vi "Add block to buffer.vi"(0 "Ring Buffer":T2, 1 "Time Stamp":timestamp, 2 "output type order":T4[](array[typedef]), 5 "data table in":T3, 7 "cache in":T1, 9 "Block size":u16, 11 "error in (no error)":errorcluster, 12 "sample counter in":i32, 13 "Pre-trigger samples?":bool) -> (4 "Ring Buffer out":T2, 6 "data table out":T3, 8 "cache out":T1, 14 "Sample counter out":i32, 15 "error out":errorcluster)   [LabVIEW 2013, in "TDMS datalogger runtime.lvclass"]
uses:
  TDMS datalogger runtime.lvclass
  data cache.ctl
  <vilib>/NI/Tag Bus/table/data table.ctl
  <vilib>/NI/Tag Bus/tag/Data Type.ctl
  Ring Buffer.ctl
  <vilib>/NI/Tag Bus/table/data table.lvlib
  <vilib>/NI/Tag Bus/tag/tag descriptor.lvclass
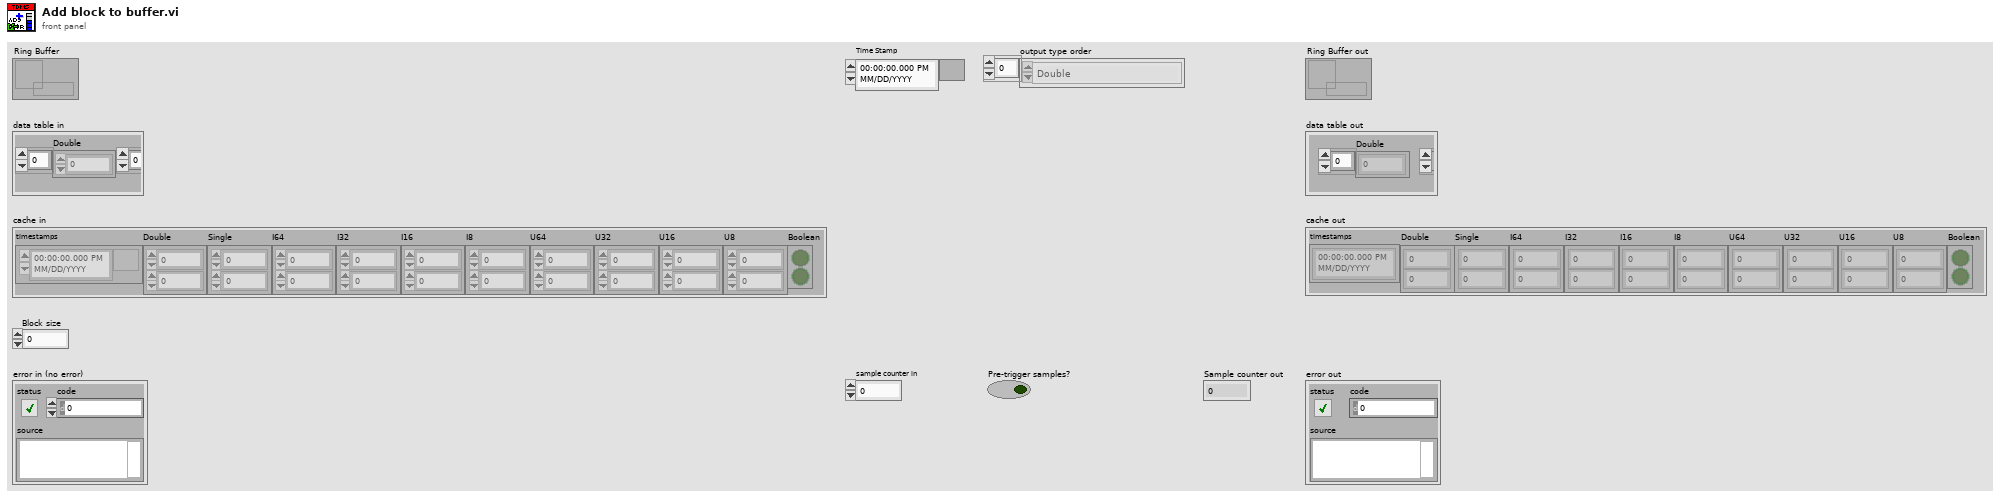
[diagram p1: front panel]
types:
  T1 = typedef "TDMS datalogger runtime.lvclass/data cache.ctl" = cluster{"timestamps":timestamp[], "Double":dbl[][], "Single":sgl[][], "I64":i64[][], "I32":i32[][], "I16":i16[][], "I8":i8[][], "U64":u64[][], "U32":u32[][], "U16":u16[][], "U8":u8[][], "Boolean":bool[][]}
  T2 = typedef "TDMS datalogger runtime.lvclass/Ring Buffer.ctl" = refnum<queue>
  T3 = typedef "tag bus.lvlib/data table.lvlib/data table.ctl" = cluster{"Double":dbl[], "Single":sgl[], "I64":i64[], "I32":i32[], "I16":i16[], "I8":i8[], "U64":u64[], "U32":u32[], "U16":u16[], "U8":u8[], "Boolean":bool[], "String":string[], "Array of Double":cluster{"DBL Array":dbl[]}[], "Array of Single":cluster{"SGL Array":sgl[]}[], "Array of I64":cluster{"I64 Array":i64[]}[], "Array of I32":cluster{"I32 Array":i32[]}[], "Array of I16":cluster{"I16 Array":i16[]}[], "Array of I8":cluster{"I8 Array":i8[]}[], "Array of U64":cluster{"U64 Array":u64[]}[], "Array of U32":cluster{"U32 Array":u32[]}[], "Array of U16":cluster{"U16 Array":u16[]}[], "Array of U8":cluster{"U8 Array":u8[]}[], "Array of Boolean":cluster{"Boolean Array":bool[]}[], "Array of String":cluster{"String Array":string[]}[]}
  T4 = typedef "tag bus.lvlib/tag descriptor.lvclass/Data Type.ctl" = enum16{"Double", "Single", "I64", "I32", "I16", "I8", "U64", "U32", "U16", "U8", "Boolean", "String", "Array of Double", "Array of Single", "Array of I64", "Array of I32", "Array of I16", "Array of I8", "Array of U64", "Array of U32", "Array of U16", "Array of U8", "Array of Boolean", "Array of String"}
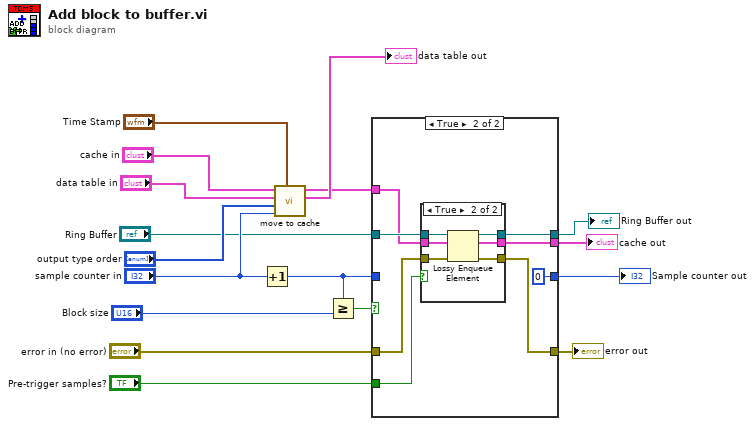
[diagram p0: block diagram]
diagram:
  n1 = Increment(x="sample counter in") -> (x+1=w2:i32)
  n2 = call "move to cache.vi"("Time Stamp"="Time Stamp", "sample counter"="sample counter in", "output type order"="output type order", "data table in"="data table in", "cache in"="cache in") -> ("data table out"=→"data table out":T3, "cache out"=w9:T1)  [unwired: 5 in]
  n3 = Greater Or Equal?(x=w2, y="Block size") -> (x >= y?=w12:bool)
  n4 = case shown="True" w12 {
    tunnel: "Ring Buffer" -> [w20 w29]
    tunnel: w9 -> [w19 w28]
    tunnel: [w20 w27] -> w8
    tunnel: [w21 w26] -> w7
    tunnel: "error in (no error)" -> [w21 w25]
    tunnel: [w19 w24] -> w4
    tunnel: "Pre-trigger samples?" -> [_ w23]
    tunnel: w2 -> [w18 _]
    tunnel: [w18 0] -> w1
    frame False {
    }
    frame True {
      n5 = case shown="True" w23 {
        tunnel: w29 -> [w31 w38]
        tunnel: w28 -> [w32 w37]
        tunnel: [w31 w36] -> w27
        tunnel: [w30 w35] -> w26
        tunnel: w25 -> [w30 w34]
        tunnel: [w32 w33] -> w24
        frame False {
        }
        frame True {
          n6 = Lossy Enqueue Element(queue=w38, element=w37, error in (no error)=w34) -> (queue out=w36:T2, overflow element=w33:T1, error out=w35:errorcluster)  [unwired: 1 out]
        }
      }
    }
  }
  "Ring Buffer out" <- w8
  "error out" <- w7
  "cache out" <- w4
  "Sample counter out" <- w1
